vi "SENS_OFFS_MULT.vi"(0 "VISA IN":refnum<visa-resource-name>, 1 "Multiplier":i32, 5 "error in":errorcluster, 7 "Channel":i32) -> (14 "VISA Out":refnum<visa-resource-name>, 19 "error out":errorcluster)   [LabVIEW 2018, in "PNA-X.lvlib"]
doc: "SENSe<cnum>:OFFSet:MULTiplier <num> \n(Read-Write) Specifies (along with the divisor) the value to multiply by the stimulus. \nParameters \n<cnum> Any existing channel number. If unspecified, value is set to 1 \n<num> Multiplier value. Range is +/- 1000. Negative multipliers cause the stimulus to \nsweep in decreasing direction. For mixer measurements, this would be for \nsetups requiring the RF frequency to be less than LO frequency \nExamples SENS:OFFS:MULT 2 \nsense2:offset:multiplier 4 \nQuery Syntax SENSe<cnum>:OFFSet:MULTplier? \nReturn Type Numeric \nDefault 1"
uses:
  PNA-X.lvlib
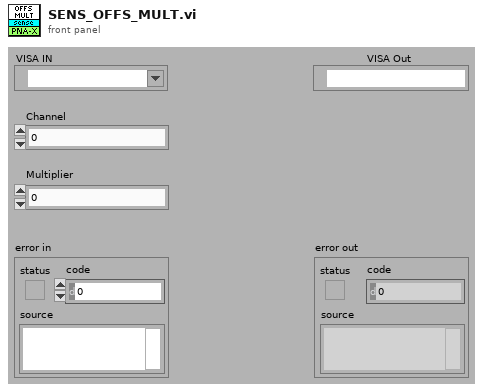
[diagram p1: front panel]
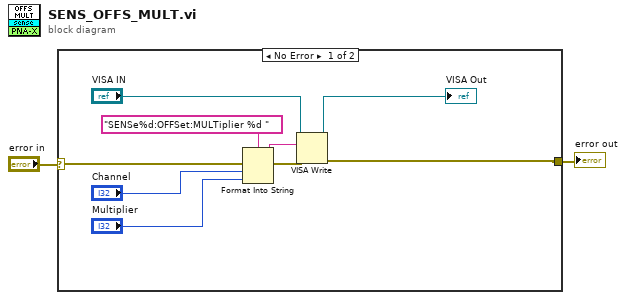
[diagram p0: block diagram]
diagram:
  n1 = case shown="No Error" "error in" {
    selector: "error in" -> [w11 w12]
    tunnel: [w6 w12] -> w1
    frame No Error {
      n2 = Format Into String(format string="SENSe%d:OFFSet:MULTiplier %d " ("Cmdline"), error in=w11, "Channel", "Multiplier") -> (resulting string=w9:string, error out=w10:errorcluster)  [unwired: 1 in]
      n3 = VISA Write(VISA resource name="VISA IN", write buffer=w9, error in (no error)=w10) -> (VISA resource name out=→"VISA Out":refnum<visa-resource-name>, error out=w6:errorcluster)  [unwired: 1 out]
    }
    frame Error {
    }
  }
  "error out" <- w1
